vi "Update Result.vi"(4 "sp time stamp":timestamp, 5 "Peaks":dbl[](array[numeric]) format="%#_4p", 6 "Good fit?":dbl[](array[numeric]) format="%#_4p", 7 "Best fit results":dbl[][](array[numeric]) format="%#_4p", 8 "error in (no error)":errorcluster, 9 "Peaks absolute time":dbl[](array[numeric]), 10 "File":refnum<class "Acquired Result.lvclass">, 11 "Resonance Detector in":refnum<class "Resonance Detector.lvclass">) -> (0 "error out":errorcluster, 2 "File out":refnum<class "Acquired Result.lvclass">, 3 "Resonance Detector out":refnum<class "Resonance Detector.lvclass">)   [LabVIEW 2020, in "Resonance Detector.lvclass"]
uses:
  Resonance Detector.lvclass
  C:/GitHub/LabActor/Process Object/Process Object.lvclass
  NHMFL_Core/Libraries/Instruments/Results/Acquired Result/Acquired Result.lvclass
  NHMFL_Core/Libraries/RUS/Fit Columns.ctl
  NHMFL_Core/Libraries/Instruments/Results/Acquired Result/Acquired Result.lvclass/Acquired Result.ctl
  Process Object/Process Object.lvclass/Process Object.ctl
  NHMFL_Core/Libraries/Instruments/Results/Acquired Result/Write Channels.vi
  NHMFL_Core/Libraries/Instruments/Results/Acquired Result/Write Group.vi
  NHMFL_Core/Libraries/Instruments/Results/Acquired Result/Write Time group.vi
  NHMFL_Core/Libraries/Instruments/Results/Acquired Result/Write Time value.vi
  Process Object/Write Result.vi
  Process Object/Write Result ready.vi
  Read Line detector configuration.vi
panel:
  # "F0         dF     Ampl   Phase   Xbgrd   Ybgrd"
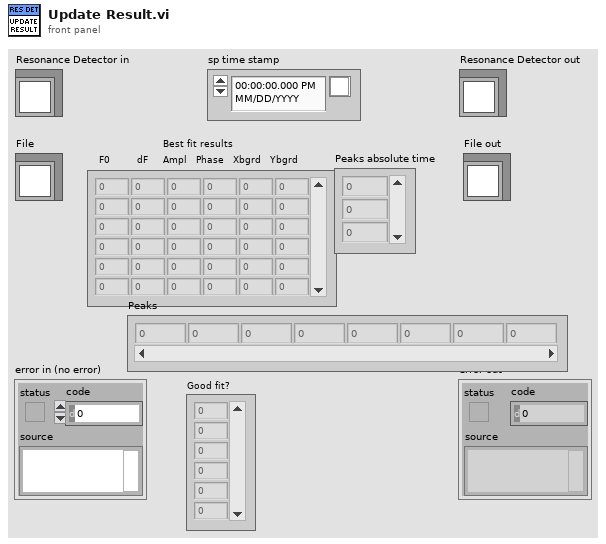
[diagram p1: front panel]
types:
  T1 = typedef "Fit Columns.ctl" = string[]
  T2 = enum16{"open", "open or create", "create or replace", "create", "open (read-only)"}
  T3 = typedef "Resonance Detector Configuration.ctl" = cluster{"Peak width guess":dbl, "Background removal":enum16{"NONE", "High-pass", "Detrend"}, "Smoothing":enum16{"NONE", "Low-pass", "Denoise"}, "Smooth window":dbl, "Relative threshold":dbl, "Finder algorithm":enum16{"Basic", "Wavelet", "Wavelet+detrend"}, "Bgd window":dbl, "Spectrum recorder module name":string, "Fit window":dbl, "Initial fit guess":enum16{"Peak finder", "Last fit"}, "Follow\npeaks":bool, "Re-sample":dbl, "Tolerance":dbl, "Max iterations":i32}
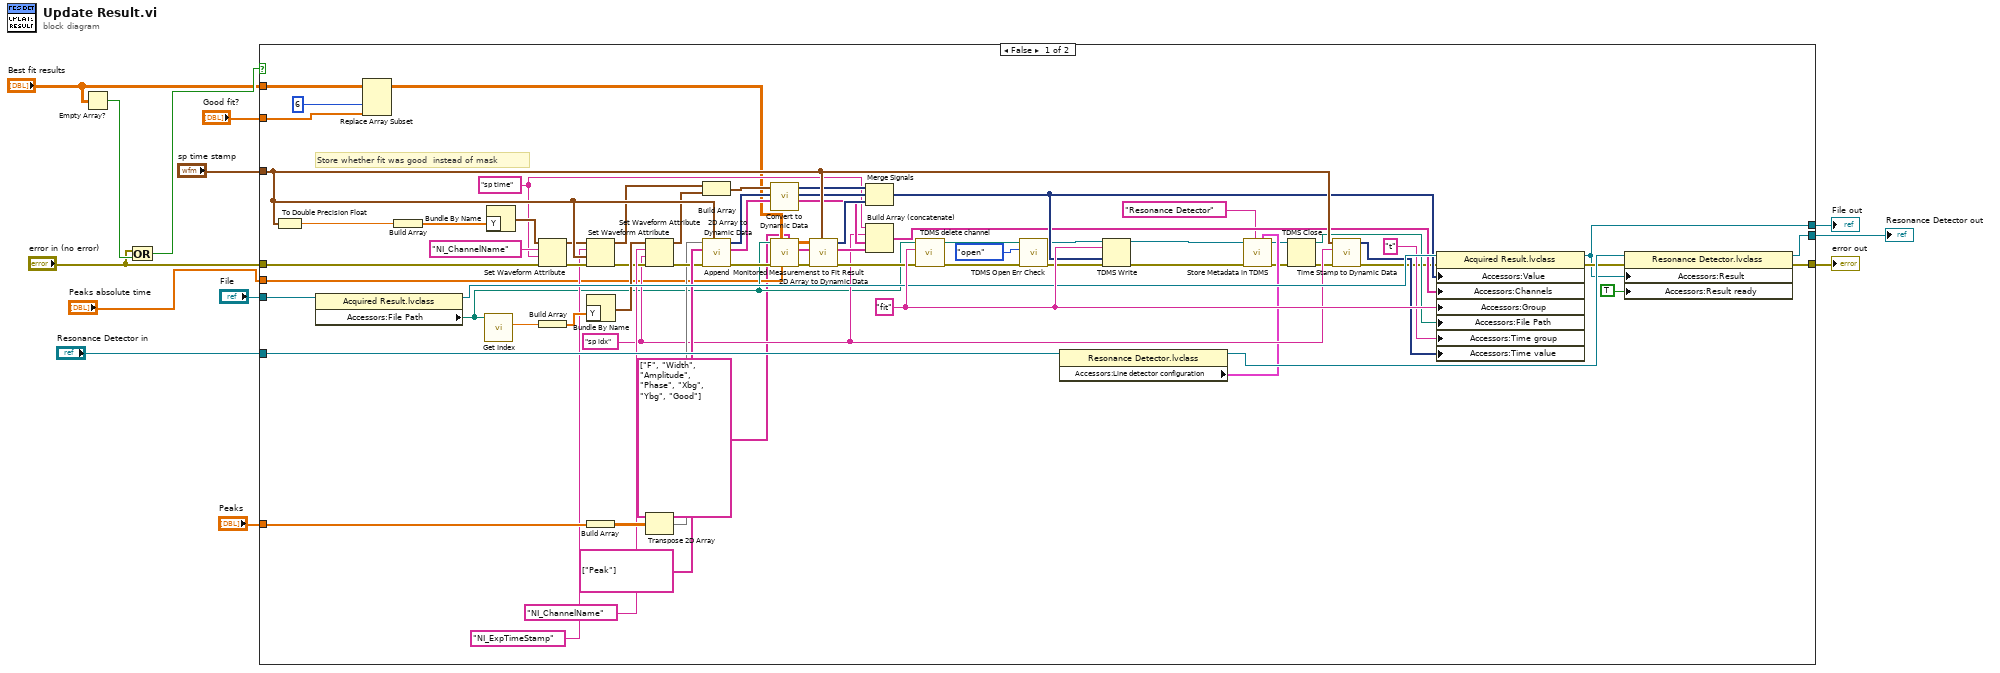
[diagram p0: block diagram]
diagram:
  n1 = Empty Array?(array="Best fit results") -> (empty?=w5:bool)
  n2 = Or(x="error in (no error)", y=w5) -> (x .or. y?=w7:bool)
  n3 = case shown="False" w7 {
    tunnel: [w33 w83] -> w13
    tunnel: [w34 w85] -> w11
    tunnel: "Resonance Detector in" -> [w78 w85]
    tunnel: "File" -> [w77 w84]
    tunnel: "Best fit results" -> [w36 _]
    tunnel: "Peaks" -> [w81 _]
    tunnel: "sp time stamp" -> [w80 _]
    tunnel: "error in (no error)" -> [w39 w83]
    tunnel: [w38 w84] -> w3
    tunnel: "Good fit?" -> [w35 _]
    tunnel: "Peaks absolute time" -> [w28 _]
    frame False {
      w57 = "sp time" ("name")
      w42 = "sp idx" ("name")
      w79 = "fit"
      # "Store whether fit was good  instead of mask"
      n4 = To Double Precision Float(number=w80) -> (double precision float=w58:dbl)
      n5 = property class="Acquired Result.lvclass"(reference=w77) -> (reference out=w76:refnum<class "Acquired Result.lvclass">, "Accessors:File Path"=w30:path)  [unwired: 1 in, 1 out]
      n6 = Replace Array Subset(array=w36, new element=w35, index (col)=6 ("disabled index (col)")) -> (w27:dbl[][])  [unwired: 1 in]
      n7 = Build Array(w58) -> (w44:dbl[])
      n8 = call "Get Index.vi"("File Path Control"=w30) -> ("DBL number"=w53:dbl)  [unwired: 9 in, 1 out]
      n9 = Bundle By Name("Y"=w44) -> (w60:waveform(dbl))  [unwired: 1 in]
      n10 = Set Waveform Attribute(4:w39, 5:w57, 6:"NI_ChannelName" ("name"), 7:w60) -> (0:w51:errorcluster, 3:w50:waveform(dbl))  [unwired: 1 out]
      n11 = Build Array(w53) -> (w69:dbl[])
      n12 = Set Waveform Attribute(4:w51, 5:w80, 6:"NI_ExpTimeStamp" ("name"), 7:w50) -> (0:w48:errorcluster, 3:w49:waveform(dbl))  [unwired: 1 out]
      n13 = Bundle By Name("Y"=w69) -> (w68:waveform(dbl))  [unwired: 1 in]
      n14 = Build Array(w81) -> (w75:dbl[][])
      n15 = Set Waveform Attribute(4:w48, 5:w42, 6:"NI_ChannelName" ("name"), 7:w68) -> (0:w66:errorcluster, 3:w45:waveform(dbl))  [unwired: 1 out]
      n16 = Transpose 2D Array(2D array=w75) -> (transposed array=w61:dbl[][])
      n17 = Build Array(w49, w45) -> (w65:waveform(dbl)[])
      n18 = call "2D Array to Dynamic Data.vi"("Time Stamp Control"=w80, "Error In"=w66, "Channels"=string[] ["Peak"], "Array"=w61) -> ("Error Out"=w32:errorcluster, "Channels out"=w71:string[], "Dynamic Data Type"=w74:dynamicdata)  [unwired: 5 in]
      n19 = call "Convert to Dynamic Data"("Array of Waveforms"=w65) -> ("Dynamic Data Type"=w64:dynamicdata)  [unwired: 3 in]
      n20 = call "Append  Monitored Measuremenst to Fit Result.vi"("Channels"=T1 ["F", "Width", "Amplitude", "Phase", "Xbg", "Ybg", "Good"], "Peaks absolute time"=w28, "Data in"=w27, "Error In"=w32, "file path"=w30) -> ("Error Out"=w31:errorcluster, "Channels out"=w29:string[], "Data out"=w26:dbl[][])  [unwired: 4 in]
      n21 = call "2D Array to Dynamic Data.vi"("Time Stamp Control"=w80, "Error In"=w31, "Channels"=w29, "Array"=w26) -> ("Error Out"=w56:errorcluster, "Channels out"=w70:string[], "Dynamic Data Type"=w73:dynamicdata)  [unwired: 5 in]
      n22 = Merge Signals(w64, w74, w73) -> (w63:dynamicdata)
      n23 = Build Array (concatenate)(w57, w42, w71, w70) -> (w62:string[])
      n24 = call "TDMS delete channel.vi"("error in (no error)"=w56, "group name"=w79, "file path"=w30) -> ("error out"=w22:errorcluster, "file path out"=w24:path)  [unwired: 6 in, 1 out]
      n25 = call "TDMS Open Err Check.vi"("Error In"=w22, "operation (0:open)"=T2."open", "File Path Control"=w24) -> ("Error Out"=w20:errorcluster, "tdms file out"=w21:refnum<k34>)  [unwired: 6 in, 1 out]
      n26 = property class="Resonance Detector.lvclass"(reference=w78) -> (reference out=w82:refnum<class "Resonance Detector.lvclass">, "Accessors:Line detector configuration"=w18:T3)  [unwired: 1 in, 1 out]
      n27 = TDMS Write(0:w21, 5:w79, 9:w63, 11:w20) -> (4:w19:refnum<k34>, 15:w16:errorcluster)  [unwired: 2 in, 2 out]
      n28 = call "Store Metadata in TDMS.vi"("Value"=w18, "name"="Resonance Detector" ("Name"), "Error In"=w16, "tdms file"=w19) -> ("Error Out"=w14:errorcluster, "tdms file out"=w15:refnum<k34>)  [unwired: 4 in, 2 out]
      n29 = TDMS Close(8:w14, 11:w15) -> (0:w41:errorcluster, 3:w54:path)
      n30 = call "Time Stamp to Dynamic Data.vi"("Error In"=w41, "Name"=w42, "Time Stamp Control"=w80) -> ("Error Out"=w40:errorcluster, "Dynamic Data Type"=w43:dynamicdata)  [unwired: 7 in]
      n31 = property class="Acquired Result.lvclass"(reference=w76, error in=w40, "Accessors:Value"=w63, "Accessors:Channels"=w62, "Accessors:Group"=w79, "Accessors:File Path"=w54, "Accessors:Time group"="t" ("Time group"), "Accessors:Time value"=w43) -> (reference out=w38:refnum<class "Acquired Result.lvclass">, error out=w55:errorcluster)
      n32 = property class="Resonance Detector.lvclass"(reference=w82, error in=w55, "Accessors:Result"=w38, "Accessors:Result ready"=TRUE ("Result ready")) -> (reference out=w34:refnum<class "Resonance Detector.lvclass">, error out=w33:errorcluster)
    }
    frame True {
    }
  }
  "error out" <- w13
  "Resonance Detector out" <- w11
  "File out" <- w3
